vi "CheckOper_45.vi"() -> ()   [LabVIEW 2012]
doc: "Required Equipment: This example assumes the following hardware configuration:\n - 34945A RF/Microwave Switch Driver in slot 1\n - 34945EXT connected to L4445A with cable\n - (1) Y1150A Distribution Module in slot 1 of 34945EXT\n - (1) N1810UL Switch in SW1 socket\n\nThis vi looks at the description of the first 34945EXT module, presets all banks on the module to default values for that distribution board type, enables verification of the switch closure (using negative polarity), closes a channel, reads the IsClosed state of that channel, and reads the drive status of the channel. (NOTE that the drive state will be \"0\" if the channel is set for Pulsed operation). NOTE also that inverted verification polarity is needed with the \nN1810UL Switch."
panel:
  in  "VISA resource name":refnum<visa-resource-name>
  out "VISA/Instrument Errors":errorcluster
  out "Is Closed?":bool[](array[boolean])
  out "Drive State":bool[](array[boolean])
  out "Remote Module Type":string
  out "Remote Module Status":string
  out "Remote Module Description":string
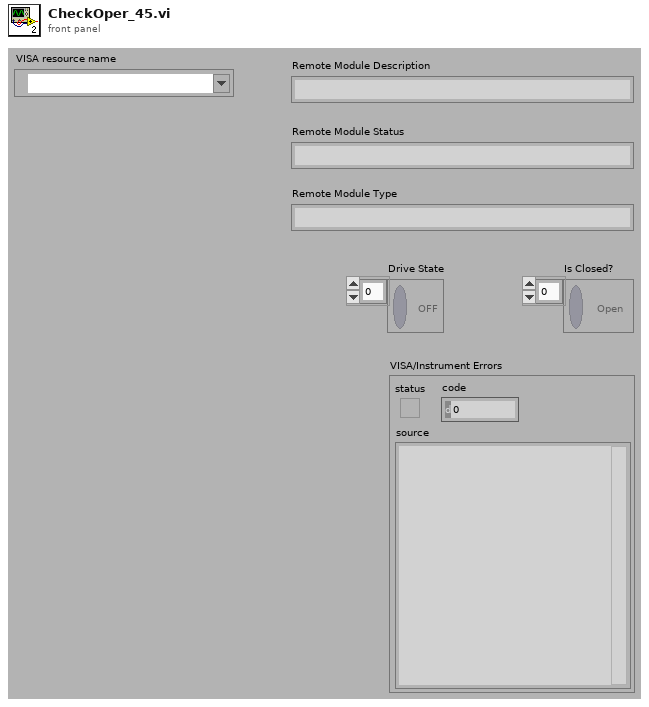
[diagram p1: front panel]
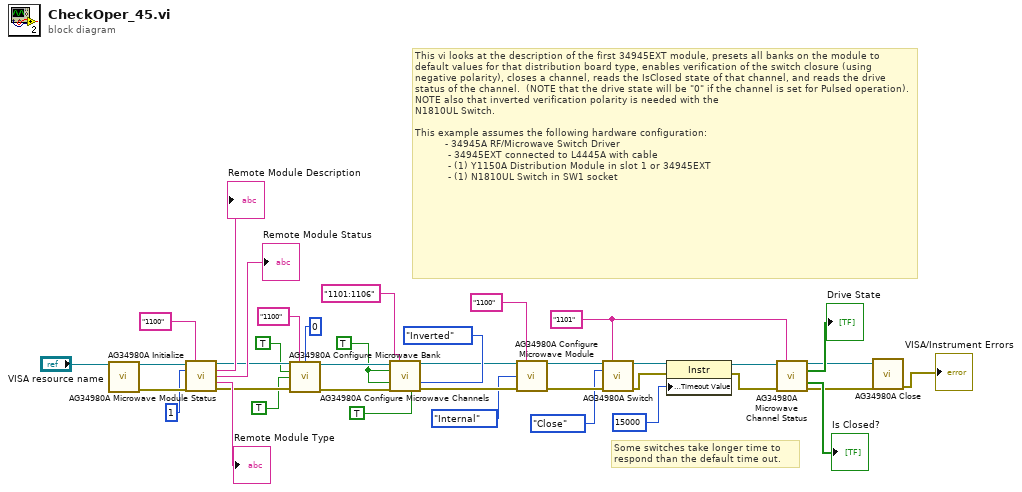
[diagram p0: block diagram]
diagram:
  w13 = "1101" ("Channel List")
  w23 = TRUE ("Disable Drive (F)")
  # "Some switches take longer time to respond than the default time out."
  # "This vi looks at the description of the first 34945EXT module, presets all banks on the module to default values for that distribution board type, enables verification of the switch closure (using negative polarity), closes a channel, reads the IsClosed state of that channel, and reads the drive status of the channel.  (NOTE that the drive state will be \"0\" if the channel is set for Pulsed operation).  NOTE also that inverted verification polarity is needed with the \nN1810UL Switch.\n\nThis example assumes the following hardware configuration:\n          - 34945A RF/Microwave Switch Driver\n           - 34945EXT connected to L4445A with cable\n           - (1) Y1150A Distribution Module in slot 1 or 34945EXT\n           - (1) N1810UL Switch in SW1 socket"
  n1 = call "AG34980A Initialize.vi"("VISA resource name"="VISA resource name") -> ("VISA session"=w38:refnum<visa-resource-name>, "error out"=w37:errorcluster)  [unwired: 13 in]
  n2 = call "AG34980A Microwave Module Status.vi"("VISA resource name"=w38, "Single Channel"="1100", "Distribution Board (-1:None)"=1, "error in (no error)"=w37) -> ("VISA resource name out"=w30:refnum<visa-resource-name>, "Remote Module Description"=→"Remote Module Description":string, "Remote Module Status"=→"Remote Module Status":string, "Remote Module Type"=→"Remote Module Type":string, "error out"=w32:errorcluster)  [unwired: 7 in]
  n3 = call "AG34980A Configure Microwave Bank.vi"("VISA resource name"=w30, "Remote Module Specifier"="1100", "Bank (0:ALL)"=0, "Disable Drive (F)"=TRUE, "Send Bank Preset (F)"=TRUE, "error in (no error)"=w32) -> ("VISA resource name out"=w26:refnum<visa-resource-name>, "error out"=w25:errorcluster)  [unwired: 8 in]
  n4 = call "AG34980A Configure Microwave Channels.vi"("VISA resource name"=w26, "Channel List"="1101:1106", "Disable Drive (F)"=w23, "Paired Mode (F)"=w23, "Verification Polarity (0:Normal)"=enum16{"Normal", "Inverted"}."Inverted", "error in (no error)"=w25, "Verification Enable (F)"=TRUE ("Pulse Mode (T)")) -> ("VISA resource name out"=w21:refnum<visa-resource-name>, "error out"=w20:errorcluster)  [unwired: 7 in]
  n5 = call "AG34980A Configure Microwave Module.vi"("VISA resource name"=w21, "Remote Module List"="1100", "Drive Source (0:Off)"=enum16{"Off", "External", "Internal"}."Internal", "error in (no error)"=w20) -> ("VISA resource name out"=w16:refnum<visa-resource-name>, "error out"=w15:errorcluster)  [unwired: 10 in]
  n6 = call "AG34980A Switch.vi"("VISA resource name"=w16, "Channel List"=w13, "Open/Close (0:Close)"=enum16{"Close", "Open"}."Close", "error in (no error)"=w15) -> ("VISA resource name out"=w4:refnum<visa-resource-name>, "error out"=w3:errorcluster)  [unwired: 9 in, 1 out]
  n7 = property class="Instr"(reference=w4, error in=w3, "General Settings:Timeout Value"=u32 15000) -> (reference out=w1:refnum<visa-resource-name>, error out=w2:errorcluster)
  n8 = call "AG34980A Microwave Channel Status.vi"("VISA resource name"=w1, "Channel List"=w13, "error in (no error)"=w2) -> ("VISA resource name out"=w10:refnum<visa-resource-name>, "Drive State"=→"Drive State":bool[], "Is Closed?"=→"Is Closed?":bool[], "error out"=w9:errorcluster)  [unwired: 9 in]
  n9 = call "AG34980A Close.vi"("VISA resource name"=w10, "error in (no error)"=w9) -> ("error out"=→"VISA/Instrument Errors":errorcluster)  [unwired: 13 in]
